vi "TextToLines.vi"(8 "error in (no error)":errorcluster, 11 "string":string) -> (0 "error out":errorcluster, 3 "Lines":string[](array[string]))   [LabVIEW 2017]
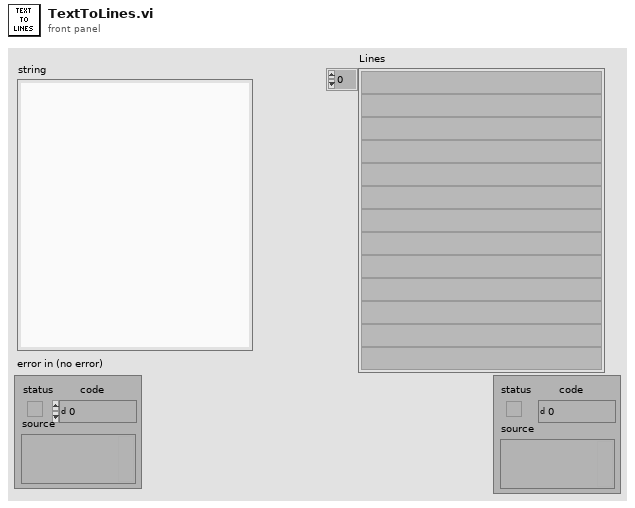
[diagram p1: front panel]
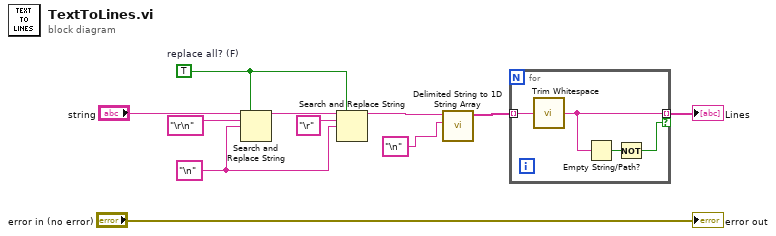
[diagram p0: block diagram]
diagram:
  w5 = TRUE  # replace all? (F)
  w6 = "\n" ("delimiter (Tab)")
  n1 = Search and Replace String(replace all?=w5, input string="string", search string="\r\n" ("delimiter (Tab)"), replace string=w6) -> (result string=w8:string)  [unwired: 4 in, 3 out]
  n2 = Search and Replace String(replace all?=w5, input string=w8, search string="\r" ("delimiter (Tab)"), replace string=w6) -> (result string=w2:string)  [unwired: 4 in, 3 out]
  n3 = call "Delimited String to 1D String Array.vi"("delimiter"="\n" ("delimiter (Tab)"), "delimited string"=w2) -> ("string array"=w9:string[])  [unwired: 9 in]
  n4 = for {
    tunnel: w9 -> [w15] mode=indexing
    tunnel: [w14] -> w10 mode=indexing if=w12
    n5 = call-poly <vilib>:"Trim Whitespace.vi"("string"=w15) -> ("trimmed string"=w14:string)  [unwired: 1 in]
    n6 = Empty String/Path?(string/path=w14) -> (empty?=w13:bool)
    n7 = Not(x=w13) -> (.not. x?=w12:bool)
  }
  "Lines" <- w10
  "error out" <- "error in (no error)"
